vi "Initialize.vi"(8 "error in (no error)":errorcluster, 9 "Reset (True)":bool=TRUE, 10 "ID Query (True)":bool=TRUE, 11 "VISA resource name":refnum<visa-resource-name>) -> (0 "error out":errorcluster, 3 "VISA resource name out":refnum<visa-resource-name>)   [LabVIEW 2020, in "Agilent B2900 Series.lvlib"]
doc: "Establishes communication with the instrument and optionally performs an instrument identification query and/or an instrument reset. It also places the instrument in a default state needed for other instrument driver operations. Therefore, call this VI before calling other instrument driver VIs for this instrument. Generally, you need to call the Initialize VI only once at the beginning of an application."
uses:
  Agilent B2900 Series.lvlib
  Private/Extended User Data.ctl
  <vilib>/regexp/Match Regular Expression.xnode
panel:
  # "(c) 2011-2021 National Instruments.  ALL RIGHTS RESERVED."
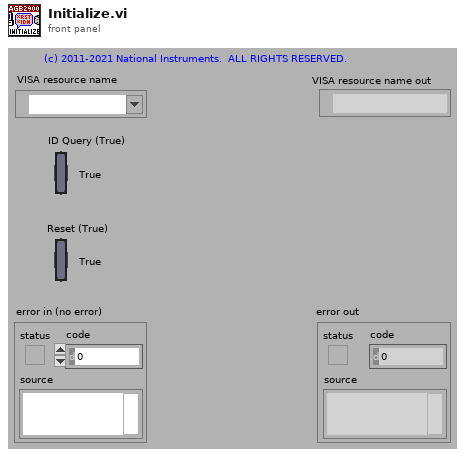
[diagram p1: front panel]
types:
  T1 = typedef "Agilent B2900 Series.lvlib/Extended User Data.ctl" = cluster{"B2900 Series Mode":u16}
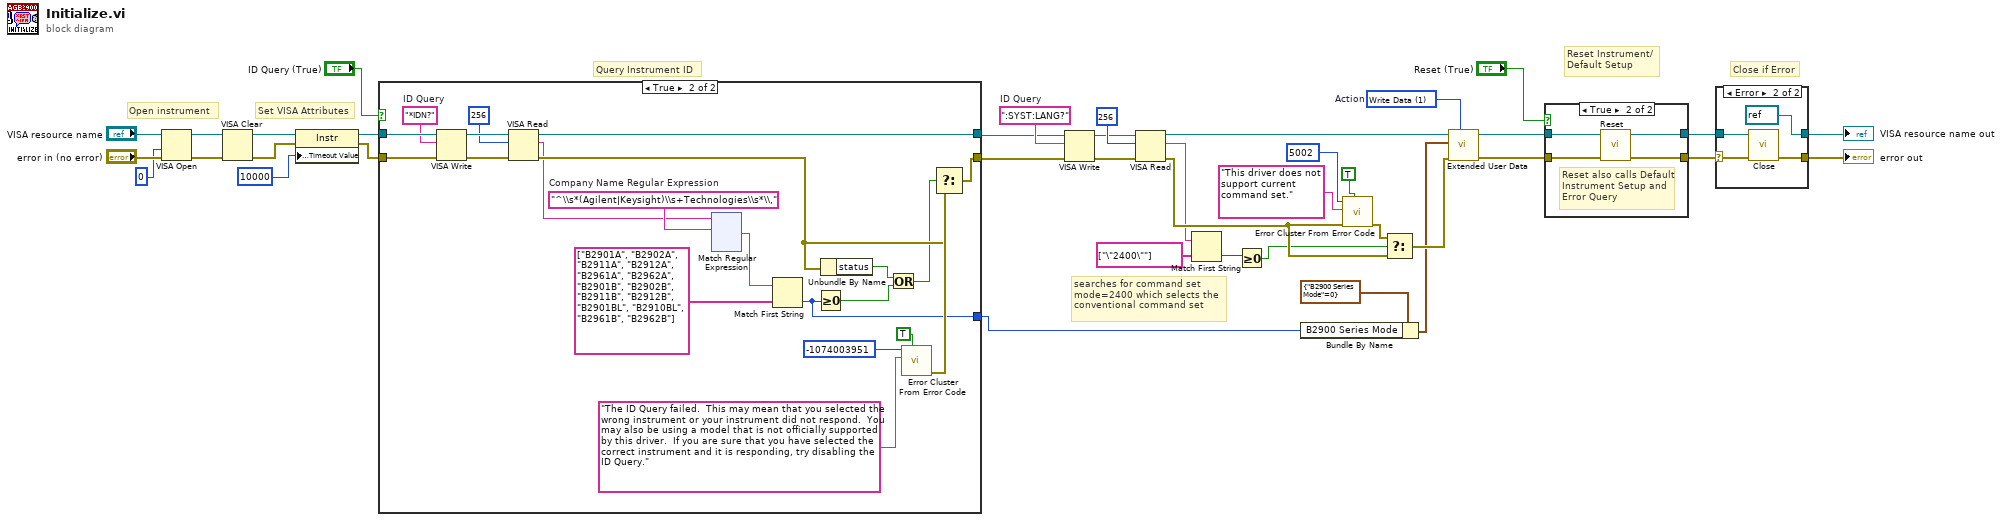
[diagram p0: block diagram]
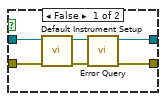
[diagram p3: hidden frame]
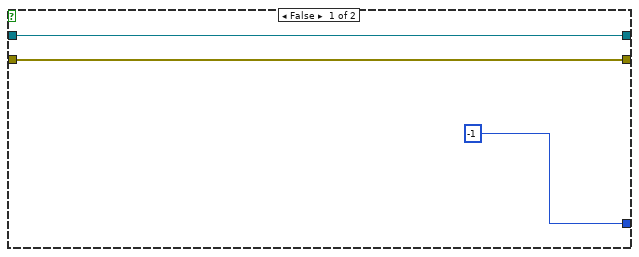
[diagram p4: hidden frame]
diagram:
  w7 = 1 items=["Read Data", "Write Data", "Clear Data", "Clear ALL Data"]  # Action
  w23 = ":SYST:LANG?"  # ID Query
  # "searches for command set \nmode=2400 which selects the\nconventional command set"
  # "Set VISA Attributes"
  # "Close if Error"
  # "Query Instrument ID"
  # "Reset Instrument/\nDefault Setup"
  # "Open instrument"
  n1 = VISA Open(access mode=u32 0, error in (no error)="error in (no error)", VISA resource name="VISA resource name") -> (VISA resource name=w33:refnum<visa-resource-name>, error out=w32:errorcluster)  [unwired: 2 in]
  n2 = VISA Clear(VISA resource name=w33, error in (no error)=w32) -> (VISA resource name out=w31:refnum<visa-resource-name>, error out=w30:errorcluster)
  n3 = property class="Instr"(reference=w31, error in=w30, "General Settings:Timeout Value"=u32 10000) -> (reference out=w25:refnum<visa-resource-name>, error out=w24:errorcluster)
  n4 = case shown="True" "ID Query (True)" {
    tunnel: [w41 w63] -> w18
    tunnel: [w42 w60] -> w19
    tunnel: w25 -> [w42 w61]
    tunnel: w24 -> [w41 w62]
    tunnel: [-1 ("index") w46] -> w8
    frame False {
    }
    frame True {
      w45 = "^\\s*(Agilent|Keysight)\\s+Technologies\\s*\\,"  # Company Name Regular Expression
      w56 = "*IDN?"  # ID Query
      n5 = VISA Write(VISA resource name=w61, write buffer=w56, error in (no error)=w62) -> (VISA resource name out=w59:refnum<visa-resource-name>, error out=w58:errorcluster)  [unwired: 1 out]
      n6 = VISA Read(VISA resource name=w59, byte count=u32 256, error in (no error)=w58) -> (VISA resource name out=w60:refnum<visa-resource-name>, read buffer=w44:string, error out=w51:errorcluster)  [unwired: 1 out]
      n7 = xnode "Match Regular Expression"("input string"=w44, "regular expression"=w45) -> ("after match"=w43:string)  [unwired: 4 in, 4 out]
      n8 = Match First String(2:string[] ["B2901A", "B2902A", "B2911A", "B2912A", "B2961A", "B2962A", "B2901B", "B2902B", "B2911B", "B2912B", "B2901BL", "B2910BL", "B2961B", "B2962B"] ("string array"), 3:w43) -> (0:w46:i32)  [unwired: 1 out]
      n9 = Greater Or Equal To 0?(x=w46) -> (x >= 0?=w49:bool)
      n10 = Unbundle By Name(w51) -> ("status"=w50:bool)
      n11 = Or(x=w50, y=w49) -> (x .or. y?=w48:bool)
      n12 = call <vilib>:"Error Cluster From Error Code.vi"("show call chain? (False)"=TRUE, "error message (\"\")"="The ID Query failed.  This may mean that you selected the wrong instrument or your instrument did not respond.  You may also be using a model that is not officially supported by this driver.  If you are sure that you have selected the correct instrument and it is responding, try disabling the ID Query." ("Source (VI Name)"), "error code (0)"=-1074003951 ("Code")) -> ("error out"=w55:errorcluster)  [unwired: 6 in]
      n13 = Select(t=w51, s=w48, f=w55) -> (s? t:f=w63:errorcluster)
    }
  }
  n14 = VISA Write(VISA resource name=w19, write buffer=w23, error in (no error)=w18) -> (VISA resource name out=w20:refnum<visa-resource-name>, error out=w21:errorcluster)  [unwired: 1 out]
  n15 = VISA Read(VISA resource name=w20, byte count=u32 256, error in (no error)=w21) -> (VISA resource name out=w5:refnum<visa-resource-name>, read buffer=w10:string, error out=w13:errorcluster)  [unwired: 1 out]
  n16 = Match First String(2:string[] ["\"2400\""] ("string array"), 3:w10) -> (0:w12:i32)  [unwired: 1 out]
  n17 = Greater Or Equal To 0?(x=w12) -> (x >= 0?=w11:bool)
  n18 = Bundle By Name(cluster=T1 {"B2900 Series Mode"=0} ("User Data In"), "B2900 Series Mode"=w8) -> (w1:T1)
  n19 = call <vilib>:"Error Cluster From Error Code.vi"("show call chain? (False)"=TRUE, "error in (no error)"=w13, "error message (\"\")"="This driver does not support current command set." ("Source (VI Name)"), "error code (0)"=5002 ("Code")) -> ("error out"=w14:errorcluster)  [unwired: 5 in]
  n20 = Select(t=w14, s=w11, f=w13) -> (s? t:f=w4:errorcluster)
  n21 = call "Extended User Data.vi"("Action (1: Write Data)"=w7, "Error In (no error)"=w4, "User Data In"=w1, "VISA resource name in"=w5) -> ("Error Out"=w3:errorcluster, "VISA resource name out"=w6:refnum<visa-resource-name>)  [unwired: 5 in, 1 out]
  n22 = case shown="True" "Reset (True)" {
    tunnel: w3 -> [w182 w184]
    tunnel: [w179 w187] -> w26
    tunnel: w6 -> [w183 w185]
    tunnel: [w180 w186] -> w27
    frame False {
      n23 = call "Default Instrument Setup.vi"("error in (no error)"=w182, "VISA resource name"=w183) -> ("error out"=w178:errorcluster, "VISA resource name out"=w181:refnum<visa-resource-name>)  [unwired: 8 in]
      n24 = call "Error Query.vi"("error in (no error)"=w178, "VISA resource name"=w181) -> ("error out"=w179:errorcluster, "VISA resource name out"=w180:refnum<visa-resource-name>)  [unwired: 6 in, 2 out]
    }
    frame True {
      # "Reset also calls Default Instrument Setup and Error Query"
      n25 = call "Reset.vi"("error in (no error)"=w184, "VISA resource name"=w185) -> ("error out"=w187:errorcluster, "VISA resource name out"=w186:refnum<visa-resource-name>)  [unwired: 8 in]
    }
  }
  n26 = case shown="Error" w26 {
    selector: w26 -> [w188 w191]
    tunnel: w27 -> [w189 w192]
    tunnel: [w189 refnum<visa-resource-name> refnum ("VISA resource name out")] -> w29
    tunnel: [w188 w193] -> w28
    frame No Error {
    }
    frame Error {
      n27 = call "Close.vi"("error in (no error)"=w191, "VISA resource name"=w192) -> ("error out"=w193:errorcluster)  [unwired: 9 in]
    }
  }
  "VISA resource name out" <- w29
  "error out" <- w28
